vi "CTRE_PigeonIMU_Receive.vi"(11 "Device ID":u32) -> (3 "Device ID Out":u32)   [LabVIEW 2016]
uses:
  <vilib>/Rock Robotics/WPI/ThirdParty/Sensors/Pigeon IMU/CTRE_PigeonIMU_CalibrationMode.ctl
  <vilib>/Rock Robotics/WPI/ThirdParty/Sensors/Pigeon IMU/CTRE_PigeonIMU_MessageIDs.ctl
  <vilib>/Rock Robotics/WPI/ThirdParty/Sensors/Pigeon IMU/CTRE_PigeonIMU_GlobalStatus.ctl
  <vilib>/Rock Robotics/WPI/ThirdParty/Sensors/Pigeon IMU/CTRE_PigeonIMU_PigeonState.ctl
  <vilib>/Rock Robotics/WPI/ThirdParty/Sensors/Pigeon IMU/CTRE_PigeonIMU_GlobalOps.ctl
panel:
  in  "CalibrationMode":T1 items=["BootTareGryoAccel"=0, "Temperature"=1, "Magnetometer12Pt"=2, "Magnetometer360"=3, "Accelerometer"=5]
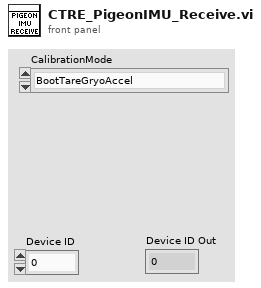
[diagram p1: front panel]
types:
  T1 = typedef "CTRE_PigeonIMU_CalibrationMode.ctl" = u16
  T2 = typedef "CTRE_PigeonIMU_MessageIDs.ctl" = u32
  T3 = typedef "CTRE_PigeonIMU_GlobalOps.ctl" = enum16{"Read For Send", "Write Error", "Get All", "Set Control Frame Rate", "Set Enable Frame Rate", "Write After Receive Fused Heading", "Write After Receive YPR", "Write After Receive Status", "Write After Receive Raw Magnetomoter", "Write After Receive Biased Magnetometer", "Write After Receive Biased Accelerometer", "Write After Receive Gyro", "Write After Receive Acceleromter Angles", "Write After Receive Startup Status", "Write After Receive Compass", "Write After Receive Quaternian", "Write After Receive AccumGyro"}
  T4 = typedef "CTRE_PigeonIMU_PigeonState.ctl" = enum16{"NoComm", "Initializing", "Ready", "UserCalibration"}
  T5 = typedef "CTRE_PigeonIMU_GlobalStatus.ctl" = cluster{"PigeonState":T4, "FusedHeading":cluster{"Heading":dbl, "Valid?":bool, "Fusing?":bool}, "YPR":cluster{"Yaw":dbl, "Pitch":dbl, "Roll":dbl}, "Compass":cluster{"Heading":dbl, "Magnitude":dbl, "Absolute Heading":dbl}, "Accelerometer":cluster{"Biased":cluster{"X":i16, "Y":i16, "Z":i16, "Norm":i16}, "Angles":cluster{"XZ Tilt":dbl, "YZ Tilt":dbl, "XY Tilt":dbl}}, "Magnetometer":cluster{"Raw":cluster{"X":i16, "Y":i16, "Z":i16}, "Biased":cluster{"X":i16, "Y":i16, "Z":i16}}, "Gyro":cluster{"X":dbl, "Y":dbl, "Z":dbl, "Norm":dbl}, "6D Quaternian":cluster{"W":dbl, "X":dbl, "Y":dbl, "Z":dbl}, "Temp. (C)":dbl, "UpTime":u32, "StartupStatus":cluster{"ResetCount":i32, "ResetFlags":i32, "FirmwareVersion":i32, "HasReset?":bool}, "Calibration":cluster{"CurrentMode":T1, "LastCalError":i32, "CalBooting?":bool}, "CAN Error":errorcluster, "AccumGyro":cluster{"X":dbl, "Y":dbl, "Z":dbl}}
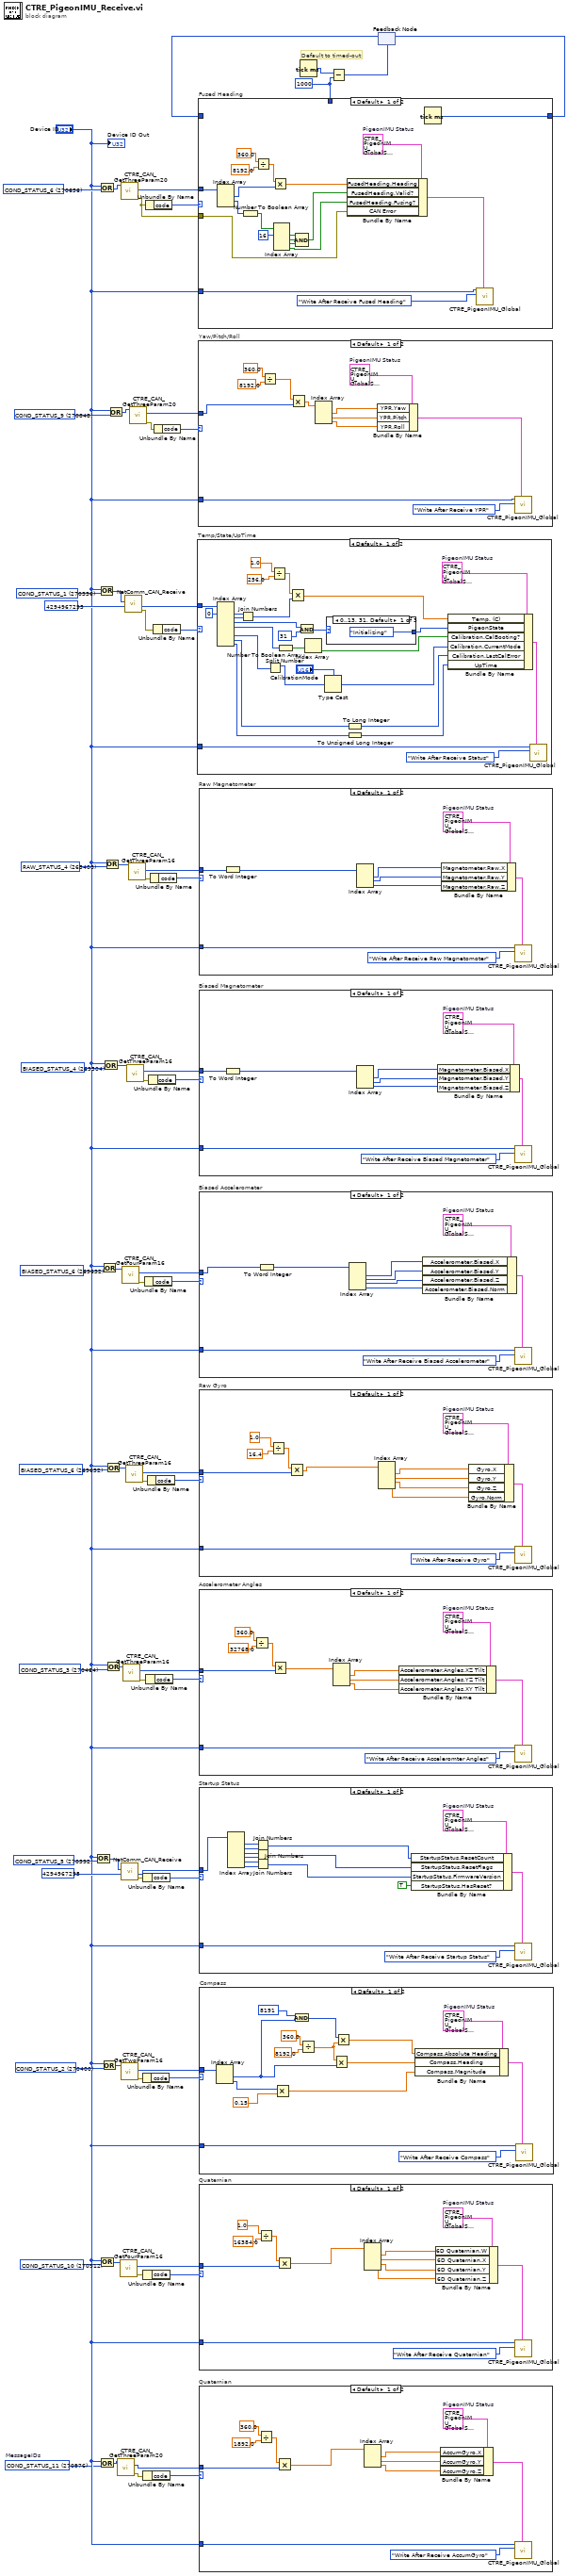
[diagram p0: block diagram]
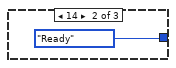
[diagram p11: hidden frame]
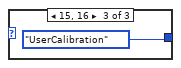
[diagram p12: hidden frame]
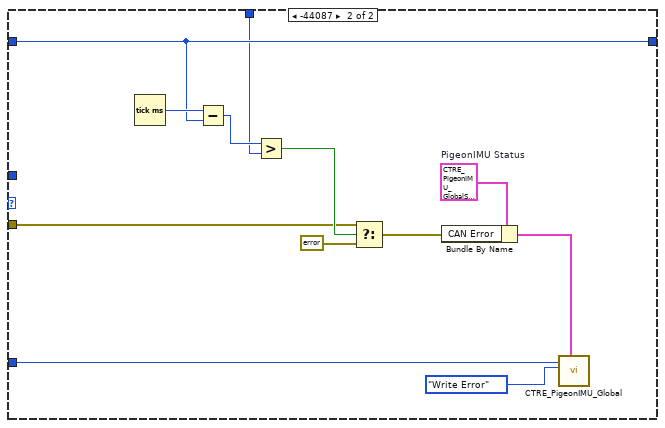
[diagram p15: hidden frame]
diagram:
  w4 = T2 270976 items=["RAW_STATUS_2"=265280, "RAW_STATUS_4"=265408, "RAW_STATUS_6"=265536, "BIASED_STATUS_2"=269376, "BIASED_STATUS_4"=269504, "BIASED_STATUS_6"=269632, "COND_STATUS_1"=270336, "COND_STATUS_2"=270400, "COND_STATUS_3"=270464, "COND_STATUS_4"=270528, "COND_STATUS_5"=270592, "COND_STATUS_6"=270656, "COND_STATUS_7"=270720, "COND_STATUS_8"=270784, "COND_STATUS_9"=270848, "COND_STATUS_10"=270912, "COND_STATUS_11"=270976, "CONTROL_1"=272384, "PARAM_REQUEST"=273408, "PARAM_RESPONSE"=273472, "PARAM_SET"=273536]  # MessageIDs
  w8 = u32 1000 ("y")
  w14 = T2 270912 items=["RAW_STATUS_2"=265280, "RAW_STATUS_4"=265408, "RAW_STATUS_6"=265536, "BIASED_STATUS_2"=269376, "BIASED_STATUS_4"=269504, "BIASED_STATUS_6"=269632, "COND_STATUS_1"=270336, "COND_STATUS_2"=270400, "COND_STATUS_3"=270464, "COND_STATUS_4"=270528, "COND_STATUS_5"=270592, "COND_STATUS_6"=270656, "COND_STATUS_7"=270720, "COND_STATUS_8"=270784, "COND_STATUS_9"=270848, "COND_STATUS_10"=270912, "CONTROL_1"=272384, "PARAM_REQUEST"=273408, "PARAM_RESPONSE"=273472, "PARAM_SET"=273536] ("MessageIDs")
  w19 = T2 270400 items=["RAW_STATUS_2"=265280, "RAW_STATUS_4"=265408, "RAW_STATUS_6"=265536, "BIASED_STATUS_2"=269376, "BIASED_STATUS_4"=269504, "BIASED_STATUS_6"=269632, "COND_STATUS_1"=270336, "COND_STATUS_2"=270400, "COND_STATUS_3"=270464, "COND_STATUS_4"=270528, "COND_STATUS_5"=270592, "COND_STATUS_6"=270656, "COND_STATUS_7"=270720, "COND_STATUS_8"=270784, "COND_STATUS_9"=270848, "COND_STATUS_10"=270912, "CONTROL_1"=272384, "PARAM_REQUEST"=273408, "PARAM_RESPONSE"=273472, "PARAM_SET"=273536] ("MessageIDs")
  w23 = T2 270592 items=["RAW_STATUS_2"=265280, "RAW_STATUS_4"=265408, "RAW_STATUS_6"=265536, "BIASED_STATUS_2"=269376, "BIASED_STATUS_4"=269504, "BIASED_STATUS_6"=269632, "COND_STATUS_1"=270336, "COND_STATUS_2"=270400, "COND_STATUS_3"=270464, "COND_STATUS_4"=270528, "COND_STATUS_5"=270592, "COND_STATUS_6"=270656, "COND_STATUS_7"=270720, "COND_STATUS_8"=270784, "COND_STATUS_9"=270848, "COND_STATUS_10"=270912, "CONTROL_1"=272384, "PARAM_REQUEST"=273408, "PARAM_RESPONSE"=273472, "PARAM_SET"=273536] ("MessageIDs")
  w31 = T2 270464 items=["RAW_STATUS_2"=265280, "RAW_STATUS_4"=265408, "RAW_STATUS_6"=265536, "BIASED_STATUS_2"=269376, "BIASED_STATUS_4"=269504, "BIASED_STATUS_6"=269632, "COND_STATUS_1"=270336, "COND_STATUS_2"=270400, "COND_STATUS_3"=270464, "COND_STATUS_4"=270528, "COND_STATUS_5"=270592, "COND_STATUS_6"=270656, "COND_STATUS_7"=270720, "COND_STATUS_8"=270784, "COND_STATUS_9"=270848, "COND_STATUS_10"=270912, "CONTROL_1"=272384, "PARAM_REQUEST"=273408, "PARAM_RESPONSE"=273472, "PARAM_SET"=273536] ("MessageIDs")
  w34 = T2 269632 items=["RAW_STATUS_2"=265280, "RAW_STATUS_4"=265408, "RAW_STATUS_6"=265536, "BIASED_STATUS_2"=269376, "BIASED_STATUS_4"=269504, "BIASED_STATUS_6"=269632, "COND_STATUS_1"=270336, "COND_STATUS_2"=270400, "COND_STATUS_3"=270464, "COND_STATUS_4"=270528, "COND_STATUS_5"=270592, "COND_STATUS_6"=270656, "COND_STATUS_7"=270720, "COND_STATUS_8"=270784, "COND_STATUS_9"=270848, "COND_STATUS_10"=270912, "CONTROL_1"=272384, "PARAM_REQUEST"=273408, "PARAM_RESPONSE"=273472, "PARAM_SET"=273536] ("MessageIDs")
  w43 = T2 269632 items=["RAW_STATUS_2"=265280, "RAW_STATUS_4"=265408, "RAW_STATUS_6"=265536, "BIASED_STATUS_2"=269376, "BIASED_STATUS_4"=269504, "BIASED_STATUS_6"=269632, "COND_STATUS_1"=270336, "COND_STATUS_2"=270400, "COND_STATUS_3"=270464, "COND_STATUS_4"=270528, "COND_STATUS_5"=270592, "COND_STATUS_6"=270656, "COND_STATUS_7"=270720, "COND_STATUS_8"=270784, "COND_STATUS_9"=270848, "COND_STATUS_10"=270912, "CONTROL_1"=272384, "PARAM_REQUEST"=273408, "PARAM_RESPONSE"=273472, "PARAM_SET"=273536] ("MessageIDs")
  w48 = T2 269504 items=["RAW_STATUS_2"=265280, "RAW_STATUS_4"=265408, "RAW_STATUS_6"=265536, "BIASED_STATUS_2"=269376, "BIASED_STATUS_4"=269504, "BIASED_STATUS_6"=269632, "COND_STATUS_1"=270336, "COND_STATUS_2"=270400, "COND_STATUS_3"=270464, "COND_STATUS_4"=270528, "COND_STATUS_5"=270592, "COND_STATUS_6"=270656, "COND_STATUS_7"=270720, "COND_STATUS_8"=270784, "COND_STATUS_9"=270848, "COND_STATUS_10"=270912, "CONTROL_1"=272384, "PARAM_REQUEST"=273408, "PARAM_RESPONSE"=273472, "PARAM_SET"=273536] ("MessageIDs")
  w49 = T2 265408 items=["RAW_STATUS_2"=265280, "RAW_STATUS_4"=265408, "RAW_STATUS_6"=265536, "BIASED_STATUS_2"=269376, "BIASED_STATUS_4"=269504, "BIASED_STATUS_6"=269632, "COND_STATUS_1"=270336, "COND_STATUS_2"=270400, "COND_STATUS_3"=270464, "COND_STATUS_4"=270528, "COND_STATUS_5"=270592, "COND_STATUS_6"=270656, "COND_STATUS_7"=270720, "COND_STATUS_8"=270784, "COND_STATUS_9"=270848, "COND_STATUS_10"=270912, "CONTROL_1"=272384, "PARAM_REQUEST"=273408, "PARAM_RESPONSE"=273472, "PARAM_SET"=273536] ("MessageIDs")
  w55 = T2 270336 items=["RAW_STATUS_2"=265280, "RAW_STATUS_4"=265408, "RAW_STATUS_6"=265536, "BIASED_STATUS_2"=269376, "BIASED_STATUS_4"=269504, "BIASED_STATUS_6"=269632, "COND_STATUS_1"=270336, "COND_STATUS_2"=270400, "COND_STATUS_3"=270464, "COND_STATUS_4"=270528, "COND_STATUS_5"=270592, "COND_STATUS_6"=270656, "COND_STATUS_7"=270720, "COND_STATUS_8"=270784, "COND_STATUS_9"=270848, "COND_STATUS_10"=270912, "CONTROL_1"=272384, "PARAM_REQUEST"=273408, "PARAM_RESPONSE"=273472, "PARAM_SET"=273536] ("MessageIDs")
  w63 = T2 270848 items=["RAW_STATUS_2"=265280, "RAW_STATUS_4"=265408, "RAW_STATUS_6"=265536, "BIASED_STATUS_2"=269376, "BIASED_STATUS_4"=269504, "BIASED_STATUS_6"=269632, "COND_STATUS_1"=270336, "COND_STATUS_2"=270400, "COND_STATUS_3"=270464, "COND_STATUS_4"=270528, "COND_STATUS_5"=270592, "COND_STATUS_6"=270656, "COND_STATUS_7"=270720, "COND_STATUS_8"=270784, "COND_STATUS_9"=270848, "COND_STATUS_10"=270912, "CONTROL_1"=272384, "PARAM_REQUEST"=273408, "PARAM_RESPONSE"=273472, "PARAM_SET"=273536] ("MessageIDs")
  w66 = T2 270656 items=["RAW_STATUS_2"=265280, "RAW_STATUS_4"=265408, "RAW_STATUS_6"=265536, "BIASED_STATUS_2"=269376, "BIASED_STATUS_4"=269504, "BIASED_STATUS_6"=269632, "COND_STATUS_1"=270336, "COND_STATUS_2"=270400, "COND_STATUS_3"=270464, "COND_STATUS_4"=270528, "COND_STATUS_5"=270592, "COND_STATUS_6"=270656, "COND_STATUS_7"=270720, "COND_STATUS_8"=270784, "COND_STATUS_9"=270848, "COND_STATUS_10"=270912, "CONTROL_1"=272384, "PARAM_REQUEST"=273408, "PARAM_RESPONSE"=273472, "PARAM_SET"=273536] ("MessageIDs")
  # "Default to timed-out"
  n1 = Or(x="Device ID", y=w23) -> (x .or. y?=w28:T2)
  n2 = Or(x="Device ID", y=w55) -> (x .or. y?=w54:T2)
  n3 = Or(x="Device ID", y=w66) -> (x .or. y?=w65:T2)
  n4 = Or(x="Device ID", y=w14) -> (x .or. y?=w15:T2)
  n5 = Or(x="Device ID", y=w4) -> (x .or. y?=w3:T2)
  n6 = Or(x="Device ID", y=w19) -> (x .or. y?=w20:T2)
  n7 = Or(x="Device ID", y=w43) -> (x .or. y?=w39:T2)
  n8 = Or(x="Device ID", y=w48) -> (x .or. y?=w47:T2)
  n9 = Or(x="Device ID", y=w49) -> (x .or. y?=w50:T2)
  n10 = Or(x="Device ID", y=w34) -> (x .or. y?=w35:T2)
  n11 = Or(x="Device ID", y=w31) -> (x .or. y?=w30:T2)
  n12 = Or(x="Device ID", y=w63) -> (x .or. y?=w64:T2)
  n13 = call <vilib>:"CTRE_CAN_GetThreeParam20.vi"("ArbID"=w3) -> ("error out"=w1:errorcluster, "3Params"=w2:i32[])  [unwired: 8 in, 1 out]
  n14 = call <vilib>:"CTRE_CAN_GetFourParam16.vi"("ArbID"=w15) -> ("error out"=w17:errorcluster, "4Params"=w13:u16[])  [unwired: 8 in, 1 out]
  n15 = call <vilib>:"CTRE_CAN_GetThreeParam20.vi"("ArbID"=w65) -> ("error out"=w7:errorcluster, "3Params"=w68:i32[])  [unwired: 8 in, 1 out]
  n16 = call <vilib>:"CTRE_CAN_GetTwoParam16.vi"("ArbID"=w20) -> ("error out"=w22:errorcluster, "2Params"=w18:u16[])  [unwired: 8 in, 1 out]
  n17 = call <vilib>:"NetComm_CAN_Receive.vi"("Message ID Mask"=u32 4294967295, "Message ID"=w28) -> ("error out"=w26:errorcluster, "Data"=w24:u8[])  [unwired: 6 in, 2 out]
  n18 = call <vilib>:"CTRE_CAN_GetFourParam16.vi"("ArbID"=w39) -> ("error out"=w40:errorcluster, "4Params"=w41:u16[])  [unwired: 8 in, 1 out]
  n19 = call <vilib>:"CTRE_CAN_GetThreeParam16.vi"("ArbID"=w30) -> ("error out"=w33:errorcluster, "3Params"=w29:u16[])  [unwired: 8 in, 1 out]
  n20 = call <vilib>:"NetComm_CAN_Receive.vi"("Message ID Mask"=u32 4294967295, "Message ID"=w54) -> ("error out"=w57:errorcluster, "Data"=w58:u8[])  [unwired: 6 in, 2 out]
  n21 = call <vilib>:"CTRE_CAN_GetThreeParam16.vi"("ArbID"=w35) -> ("error out"=w37:errorcluster, "3Params"=w36:u16[])  [unwired: 8 in, 1 out]
  n22 = call <vilib>:"CTRE_CAN_GetThreeParam16.vi"("ArbID"=w47) -> ("error out"=w46:errorcluster, "3Params"=w44:u16[])  [unwired: 8 in, 1 out]
  n23 = call <vilib>:"CTRE_CAN_GetThreeParam16.vi"("ArbID"=w50) -> ("error out"=w53:errorcluster, "3Params"=w51:u16[])  [unwired: 8 in, 1 out]
  n24 = call <vilib>:"CTRE_CAN_GetThreeParam20.vi"("ArbID"=w64) -> ("error out"=w62:errorcluster, "3Params"=w60:i32[])  [unwired: 8 in, 1 out]
  n25 = Unbundle By Name(w22) -> ("code"=w21:i32)
  n26 = Unbundle By Name(w26) -> ("code"=w25:i32)
  n27 = Unbundle By Name(w17) -> ("code"=w16:i32)
  n28 = Unbundle By Name(w1) -> ("code"=w6:i32)
  n29 = Unbundle By Name(w40) -> ("code"=w42:i32)
  n30 = Unbundle By Name(w7) -> ("code"=w67:i32)
  n31 = Unbundle By Name(w33) -> ("code"=w32:i32)
  n32 = Unbundle By Name(w37) -> ("code"=w38:i32)
  n33 = Unbundle By Name(w46) -> ("code"=w45:i32)
  n34 = Unbundle By Name(w53) -> ("code"=w52:i32)
  n35 = Unbundle By Name(w57) -> ("code"=w56:i32)
  n36 = Unbundle By Name(w62) -> ("code"=w61:i32)
  n37 = case "Temp/State/UpTime" shown="Default" w56 {
    tunnel: w58 -> [w93 _]
    tunnel: "Device ID" -> [w81 _]
    frame Default {
      w95 = T5 {"PigeonState"=enum."NoComm", "FusedHeading"={"Heading"=0.0, "Valid?"=TRUE, "Fusing?"=TRUE}, "YPR"={"Yaw"=0.0, "Pitch"=0.0, "Roll"=0.0}, "Compass"={"Heading"=0.0, "Magnitude"=0.0, "Absolute Heading"=0.0}, "Accelerometer"={"Biased"={"X"=0, "Y"=0, "Z"=0, "Norm"=0}, "Angles"={"XZ Tilt"=0.0, "YZ Tilt"=0.0, "XY Tilt"=0.0}}, "Magnetometer"={"Raw"={"X"=0, "Y"=0, "Z"=0}, "Biased"={"X"=0, "Y"=0, "Z"=0}}, "Gyro"={"X"=0.0, "Y"=0.0, "Z"=0.0, "Norm"=0.0}, "6D Quaternian"={"W"=0.0, "X"=0.0, "Y"=0.0, "Z"=0.0}, "Temp. (C)"=0.0, "UpTime"=0, "StartupStatus"={"ResetCount"=0, "ResetFlags"=0, "FirmwareVersion"=0, "HasReset?"=TRUE}, "Calibration"={"CurrentMode"=0, "LastCalError"=0, "CalBooting?"=TRUE}, "CAN Error"={"status"=FALSE, "code"=0, "source"=""}, "AccumGyro"={"X"=0.0, "Y"=0.0, "Z"=0.0}}  # PigeonIMU Status
      n38 = Index Array(array=w93, index #1=0 ("index")) -> (element #1=w92:u8, element #2=w91:u8, element #3=w90:u8, element #4=w75:u8, element #6=w72:u8, element #7=w77:u8, element #8=w78:u8)  [unwired: 7 in, 1 out]
      n39 = Join Numbers(hi=w92, lo=w91) -> ((hi.lo)=w84:u16)
      n40 = Split Number(x=w72) -> (hi(x)=w71:u8)  [unwired: 1 out]
      n41 = Divide(x=1.0, y=256.0) -> (x/y=w85:dbl)
      n42 = Number To Boolean Array(number=w75) -> (Boolean array=w74:bool[])
      n43 = Multiply(x=w85, y=w84) -> (x*y=w83:dbl)
      n44 = And(x=w90, y=u8 31) -> (x .and. y?=w89:u8)
      n45 = Index Array(array=w74) -> (element=w73:bool)  [unwired: 1 in]
      n46 = Type Cast(type="CalibrationMode", x=w71) -> (*(type *) &x=w69:T1)
      n47 = case shown="0..13, 31, Default" w89 {
        tunnel: [CTRE_PigeonIMU_PigeonState."Initializing" ("PigeonState") CTRE_PigeonIMU_PigeonState."Ready" ("PigeonState") CTRE_PigeonIMU_PigeonState."UserCalibration" ("PigeonState")] -> w88
        frame 0..13, 31, Default {
        }
        frame 14 {
        }
        frame 15, 16 {
        }
      }
      n48 = To Long Integer(number=w77) -> (32bit integer=w79:i32)
      n49 = To Unsigned Long Integer(number=w78) -> (unsigned 32bit integer=w80:u32)
      n50 = Bundle By Name(cluster=w95, "Temp. (C)"=w83, "PigeonState"=w88, "Calibration.CalBooting?"=w73, "Calibration.CurrentMode"=w69, "Calibration.LastCalError"=w79, "UpTime"=w80) -> (w94:T5)
      n51 = call <vilib>:"CTRE_PigeonIMU_Global.vi"("Write After Receive"=w94, "Operation"=CTRE_PigeonIMU_GlobalOps."Write After Receive Status", "Device ID (0)"=w81) -> ()  [unwired: 6 in, 3 out]
    }
    frame -44087 {
    }
  }
  n52 = case "Yaw/Pitch/Roll" shown="Default" w61 {
    tunnel: w60 -> [w101 _]
    tunnel: "Device ID" -> [w100 _]
    frame Default {
      w110 = T5 {"PigeonState"=enum."NoComm", "FusedHeading"={"Heading"=0.0, "Valid?"=TRUE, "Fusing?"=TRUE}, "YPR"={"Yaw"=0.0, "Pitch"=0.0, "Roll"=0.0}, "Compass"={"Heading"=0.0, "Magnitude"=0.0, "Absolute Heading"=0.0}, "Accelerometer"={"Biased"={"X"=0, "Y"=0, "Z"=0, "Norm"=0}, "Angles"={"XZ Tilt"=0.0, "YZ Tilt"=0.0, "XY Tilt"=0.0}}, "Magnetometer"={"Raw"={"X"=0, "Y"=0, "Z"=0}, "Biased"={"X"=0, "Y"=0, "Z"=0}}, "Gyro"={"X"=0.0, "Y"=0.0, "Z"=0.0, "Norm"=0.0}, "6D Quaternian"={"W"=0.0, "X"=0.0, "Y"=0.0, "Z"=0.0}, "Temp. (C)"=0.0, "UpTime"=0, "StartupStatus"={"ResetCount"=0, "ResetFlags"=0, "FirmwareVersion"=0, "HasReset?"=TRUE}, "Calibration"={"CurrentMode"=0, "LastCalError"=0, "CalBooting?"=TRUE}, "CAN Error"={"status"=FALSE, "code"=0, "source"=""}, "AccumGyro"={"X"=0.0, "Y"=0.0, "Z"=0.0}}  # PigeonIMU Status
      n53 = Divide(x=360.0, y=8192.0) -> (x/y=w106:dbl)
      n54 = Multiply(x=w106, y=w101) -> (x*y=w105:dbl[])
      n55 = Index Array(array=w105) -> (element #1=w104:dbl, element #2=w103:dbl, element #3=w102:dbl)  [unwired: 3 in]
      n56 = Bundle By Name(cluster=w110, "YPR.Yaw"=w104, "YPR.Pitch"=w103, "YPR.Roll"=w102) -> (w109:T5)
      n57 = call <vilib>:"CTRE_PigeonIMU_Global.vi"("Write After Receive"=w109, "Operation"=CTRE_PigeonIMU_GlobalOps."Write After Receive YPR", "Device ID (0)"=w100) -> ()  [unwired: 6 in, 3 out]
    }
    frame -44087 {
    }
  }
  n58 = case "Raw Magnetometer" shown="Default" w52 {
    tunnel: w51 -> [w117 _]
    tunnel: "Device ID" -> [w112 _]
    frame Default {
      w119 = T5 {"PigeonState"=enum."NoComm", "FusedHeading"={"Heading"=0.0, "Valid?"=TRUE, "Fusing?"=TRUE}, "YPR"={"Yaw"=0.0, "Pitch"=0.0, "Roll"=0.0}, "Compass"={"Heading"=0.0, "Magnitude"=0.0, "Absolute Heading"=0.0}, "Accelerometer"={"Biased"={"X"=0, "Y"=0, "Z"=0, "Norm"=0}, "Angles"={"XZ Tilt"=0.0, "YZ Tilt"=0.0, "XY Tilt"=0.0}}, "Magnetometer"={"Raw"={"X"=0, "Y"=0, "Z"=0}, "Biased"={"X"=0, "Y"=0, "Z"=0}}, "Gyro"={"X"=0.0, "Y"=0.0, "Z"=0.0, "Norm"=0.0}, "6D Quaternian"={"W"=0.0, "X"=0.0, "Y"=0.0, "Z"=0.0}, "Temp. (C)"=0.0, "UpTime"=0, "StartupStatus"={"ResetCount"=0, "ResetFlags"=0, "FirmwareVersion"=0, "HasReset?"=TRUE}, "Calibration"={"CurrentMode"=0, "LastCalError"=0, "CalBooting?"=TRUE}, "CAN Error"={"status"=FALSE, "code"=0, "source"=""}, "AccumGyro"={"X"=0.0, "Y"=0.0, "Z"=0.0}}  # PigeonIMU Status
      n59 = To Word Integer(number=w117) -> (16bit integer=w113:i16[])
      n60 = Index Array(array=w113) -> (element #1=w116:i16, element #2=w115:i16, element #3=w114:i16)  [unwired: 3 in]
      n61 = Bundle By Name(cluster=w119, "Magnetometer.Raw.X"=w116, "Magnetometer.Raw.Y"=w115, "Magnetometer.Raw.Z"=w114) -> (w118:T5)
      n62 = call <vilib>:"CTRE_PigeonIMU_Global.vi"("Write After Receive"=w118, "Operation"=CTRE_PigeonIMU_GlobalOps."Write After Receive Raw Magnetomoter", "Device ID (0)"=w112) -> ()  [unwired: 6 in, 3 out]
    }
    frame -44087 {
    }
  }
  n63 = case "Biased Magnetometer" shown="Default" w45 {
    tunnel: w44 -> [w126 _]
    tunnel: "Device ID" -> [w121 _]
    frame Default {
      w128 = T5 {"PigeonState"=enum."NoComm", "FusedHeading"={"Heading"=0.0, "Valid?"=TRUE, "Fusing?"=TRUE}, "YPR"={"Yaw"=0.0, "Pitch"=0.0, "Roll"=0.0}, "Compass"={"Heading"=0.0, "Magnitude"=0.0, "Absolute Heading"=0.0}, "Accelerometer"={"Biased"={"X"=0, "Y"=0, "Z"=0, "Norm"=0}, "Angles"={"XZ Tilt"=0.0, "YZ Tilt"=0.0, "XY Tilt"=0.0}}, "Magnetometer"={"Raw"={"X"=0, "Y"=0, "Z"=0}, "Biased"={"X"=0, "Y"=0, "Z"=0}}, "Gyro"={"X"=0.0, "Y"=0.0, "Z"=0.0, "Norm"=0.0}, "6D Quaternian"={"W"=0.0, "X"=0.0, "Y"=0.0, "Z"=0.0}, "Temp. (C)"=0.0, "UpTime"=0, "StartupStatus"={"ResetCount"=0, "ResetFlags"=0, "FirmwareVersion"=0, "HasReset?"=TRUE}, "Calibration"={"CurrentMode"=0, "LastCalError"=0, "CalBooting?"=TRUE}, "CAN Error"={"status"=FALSE, "code"=0, "source"=""}, "AccumGyro"={"X"=0.0, "Y"=0.0, "Z"=0.0}}  # PigeonIMU Status
      n64 = To Word Integer(number=w126) -> (16bit integer=w122:i16[])
      n65 = Index Array(array=w122) -> (element #1=w125:i16, element #2=w124:i16, element #3=w123:i16)  [unwired: 3 in]
      n66 = Bundle By Name(cluster=w128, "Magnetometer.Biased.X"=w125, "Magnetometer.Biased.Y"=w124, "Magnetometer.Biased.Z"=w123) -> (w127:T5)
      n67 = call <vilib>:"CTRE_PigeonIMU_Global.vi"("Write After Receive"=w127, "Operation"=CTRE_PigeonIMU_GlobalOps."Write After Receive Biased Magnetometer", "Device ID (0)"=w121) -> ()  [unwired: 6 in, 3 out]
    }
    frame -44087 {
    }
  }
  n68 = case "Biased Accelerometer" shown="Default" w42 {
    tunnel: w41 -> [w136 _]
    tunnel: "Device ID" -> [w130 _]
    frame Default {
      w138 = T5 {"PigeonState"=enum."NoComm", "FusedHeading"={"Heading"=0.0, "Valid?"=TRUE, "Fusing?"=TRUE}, "YPR"={"Yaw"=0.0, "Pitch"=0.0, "Roll"=0.0}, "Compass"={"Heading"=0.0, "Magnitude"=0.0, "Absolute Heading"=0.0}, "Accelerometer"={"Biased"={"X"=0, "Y"=0, "Z"=0, "Norm"=0}, "Angles"={"XZ Tilt"=0.0, "YZ Tilt"=0.0, "XY Tilt"=0.0}}, "Magnetometer"={"Raw"={"X"=0, "Y"=0, "Z"=0}, "Biased"={"X"=0, "Y"=0, "Z"=0}}, "Gyro"={"X"=0.0, "Y"=0.0, "Z"=0.0, "Norm"=0.0}, "6D Quaternian"={"W"=0.0, "X"=0.0, "Y"=0.0, "Z"=0.0}, "Temp. (C)"=0.0, "UpTime"=0, "StartupStatus"={"ResetCount"=0, "ResetFlags"=0, "FirmwareVersion"=0, "HasReset?"=TRUE}, "Calibration"={"CurrentMode"=0, "LastCalError"=0, "CalBooting?"=TRUE}, "CAN Error"={"status"=FALSE, "code"=0, "source"=""}, "AccumGyro"={"X"=0.0, "Y"=0.0, "Z"=0.0}}  # PigeonIMU Status
      n69 = To Word Integer(number=w136) -> (16bit integer=w131:i16[])
      n70 = Index Array(array=w131) -> (element #1=w135:i16, element #2=w134:i16, element #3=w133:i16, element #4=w132:i16)  [unwired: 4 in]
      n71 = Bundle By Name(cluster=w138, "Accelerometer.Biased.X"=w135, "Accelerometer.Biased.Y"=w134, "Accelerometer.Biased.Z"=w133, "Accelerometer.Biased.Norm"=w132) -> (w137:T5)
      n72 = call <vilib>:"CTRE_PigeonIMU_Global.vi"("Write After Receive"=w137, "Operation"=CTRE_PigeonIMU_GlobalOps."Write After Receive Biased Accelerometer", "Device ID (0)"=w130) -> ()  [unwired: 6 in, 3 out]
    }
    frame -44087 {
    }
  }
  n73 = case "Raw Gyro" shown="Default" w38 {
    tunnel: w36 -> [w146 _]
    tunnel: "Device ID" -> [w140 _]
    frame Default {
      w151 = T5 {"PigeonState"=enum."NoComm", "FusedHeading"={"Heading"=0.0, "Valid?"=TRUE, "Fusing?"=TRUE}, "YPR"={"Yaw"=0.0, "Pitch"=0.0, "Roll"=0.0}, "Compass"={"Heading"=0.0, "Magnitude"=0.0, "Absolute Heading"=0.0}, "Accelerometer"={"Biased"={"X"=0, "Y"=0, "Z"=0, "Norm"=0}, "Angles"={"XZ Tilt"=0.0, "YZ Tilt"=0.0, "XY Tilt"=0.0}}, "Magnetometer"={"Raw"={"X"=0, "Y"=0, "Z"=0}, "Biased"={"X"=0, "Y"=0, "Z"=0}}, "Gyro"={"X"=0.0, "Y"=0.0, "Z"=0.0, "Norm"=0.0}, "6D Quaternian"={"W"=0.0, "X"=0.0, "Y"=0.0, "Z"=0.0}, "Temp. (C)"=0.0, "UpTime"=0, "StartupStatus"={"ResetCount"=0, "ResetFlags"=0, "FirmwareVersion"=0, "HasReset?"=TRUE}, "Calibration"={"CurrentMode"=0, "LastCalError"=0, "CalBooting?"=TRUE}, "CAN Error"={"status"=FALSE, "code"=0, "source"=""}, "AccumGyro"={"X"=0.0, "Y"=0.0, "Z"=0.0}}  # PigeonIMU Status
      n74 = Divide(x=1.0, y=16.4) -> (x/y=w147:dbl)
      n75 = Multiply(x=w147, y=w146) -> (x*y=w145:dbl[])
      n76 = Index Array(array=w145) -> (element #1=w144:dbl, element #2=w143:dbl, element #3=w142:dbl, element #4=w141:dbl)  [unwired: 4 in]
      n77 = Bundle By Name(cluster=w151, "Gyro.X"=w144, "Gyro.Y"=w143, "Gyro.Z"=w142, "Gyro.Norm"=w141) -> (w150:T5)
      n78 = call <vilib>:"CTRE_PigeonIMU_Global.vi"("Write After Receive"=w150, "Operation"=CTRE_PigeonIMU_GlobalOps."Write After Receive Gyro", "Device ID (0)"=w140) -> ()  [unwired: 6 in, 3 out]
    }
    frame -44087 {
    }
  }
  n79 = case "Accelerometer Angles" shown="Default" w32 {
    tunnel: w29 -> [w158 _]
    tunnel: "Device ID" -> [w153 _]
    frame Default {
      w163 = T5 {"PigeonState"=enum."NoComm", "FusedHeading"={"Heading"=0.0, "Valid?"=TRUE, "Fusing?"=TRUE}, "YPR"={"Yaw"=0.0, "Pitch"=0.0, "Roll"=0.0}, "Compass"={"Heading"=0.0, "Magnitude"=0.0, "Absolute Heading"=0.0}, "Accelerometer"={"Biased"={"X"=0, "Y"=0, "Z"=0, "Norm"=0}, "Angles"={"XZ Tilt"=0.0, "YZ Tilt"=0.0, "XY Tilt"=0.0}}, "Magnetometer"={"Raw"={"X"=0, "Y"=0, "Z"=0}, "Biased"={"X"=0, "Y"=0, "Z"=0}}, "Gyro"={"X"=0.0, "Y"=0.0, "Z"=0.0, "Norm"=0.0}, "6D Quaternian"={"W"=0.0, "X"=0.0, "Y"=0.0, "Z"=0.0}, "Temp. (C)"=0.0, "UpTime"=0, "StartupStatus"={"ResetCount"=0, "ResetFlags"=0, "FirmwareVersion"=0, "HasReset?"=TRUE}, "Calibration"={"CurrentMode"=0, "LastCalError"=0, "CalBooting?"=TRUE}, "CAN Error"={"status"=FALSE, "code"=0, "source"=""}, "AccumGyro"={"X"=0.0, "Y"=0.0, "Z"=0.0}}  # PigeonIMU Status
      n80 = Divide(x=360.0, y=32768.0) -> (x/y=w161:dbl)
      n81 = Multiply(x=w161, y=w158) -> (x*y=w157:dbl[])
      n82 = Index Array(array=w157) -> (element #1=w156:dbl, element #2=w155:dbl, element #3=w154:dbl)  [unwired: 3 in]
      n83 = Bundle By Name(cluster=w163, "Accelerometer.Angles.XZ Tilt"=w156, "Accelerometer.Angles.YZ Tilt"=w155, "Accelerometer.Angles.XY Tilt"=w154) -> (w162:T5)
      n84 = call <vilib>:"CTRE_PigeonIMU_Global.vi"("Write After Receive"=w162, "Operation"=CTRE_PigeonIMU_GlobalOps."Write After Receive Acceleromter Angles", "Device ID (0)"=w153) -> ()  [unwired: 6 in, 3 out]
    }
    frame -44087 {
    }
  }
  n85 = case "Startup Status" shown="Default" w25 {
    tunnel: w24 -> [w175 _]
    tunnel: "Device ID" -> [w165 _]
    frame Default {
      w178 = T5 {"PigeonState"=enum."NoComm", "FusedHeading"={"Heading"=0.0, "Valid?"=TRUE, "Fusing?"=TRUE}, "YPR"={"Yaw"=0.0, "Pitch"=0.0, "Roll"=0.0}, "Compass"={"Heading"=0.0, "Magnitude"=0.0, "Absolute Heading"=0.0}, "Accelerometer"={"Biased"={"X"=0, "Y"=0, "Z"=0, "Norm"=0}, "Angles"={"XZ Tilt"=0.0, "YZ Tilt"=0.0, "XY Tilt"=0.0}}, "Magnetometer"={"Raw"={"X"=0, "Y"=0, "Z"=0}, "Biased"={"X"=0, "Y"=0, "Z"=0}}, "Gyro"={"X"=0.0, "Y"=0.0, "Z"=0.0, "Norm"=0.0}, "6D Quaternian"={"W"=0.0, "X"=0.0, "Y"=0.0, "Z"=0.0}, "Temp. (C)"=0.0, "UpTime"=0, "StartupStatus"={"ResetCount"=0, "ResetFlags"=0, "FirmwareVersion"=0, "HasReset?"=TRUE}, "Calibration"={"CurrentMode"=0, "LastCalError"=0, "CalBooting?"=TRUE}, "CAN Error"={"status"=FALSE, "code"=0, "source"=""}, "AccumGyro"={"X"=0.0, "Y"=0.0, "Z"=0.0}}  # PigeonIMU Status
      n86 = Index Array(array=w175) -> (element #1=w173:u8, element #2=w174:u8, element #3=w170:u8, element #4=w171:u8, element #5=w168:u8, element #6=w167:u8)  [unwired: 6 in]
      n87 = Join Numbers(hi=w173, lo=w174) -> ((hi.lo)=w172:u16)
      n88 = Join Numbers(hi=w170, lo=w171) -> ((hi.lo)=w169:u16)
      n89 = Join Numbers(hi=w168, lo=w167) -> ((hi.lo)=w166:u16)
      n90 = Bundle By Name(cluster=w178, "StartupStatus.ResetCount"=w172, "StartupStatus.ResetFlags"=w169, "StartupStatus.FirmwareVersion"=w166, "StartupStatus.HasReset?"=TRUE) -> (w177:T5)
      n91 = call <vilib>:"CTRE_PigeonIMU_Global.vi"("Write After Receive"=w177, "Operation"=CTRE_PigeonIMU_GlobalOps."Write After Receive Startup Status", "Device ID (0)"=w165) -> ()  [unwired: 6 in, 3 out]
    }
    frame -44087 {
    }
  }
  n92 = case "Quaternian" shown="Default" w16 {
    tunnel: w13 -> [w186 _]
    tunnel: "Device ID" -> [w180 _]
    frame Default {
      w191 = T5 {"PigeonState"=enum."NoComm", "FusedHeading"={"Heading"=0.0, "Valid?"=TRUE, "Fusing?"=TRUE}, "YPR"={"Yaw"=0.0, "Pitch"=0.0, "Roll"=0.0}, "Compass"={"Heading"=0.0, "Magnitude"=0.0, "Absolute Heading"=0.0}, "Accelerometer"={"Biased"={"X"=0, "Y"=0, "Z"=0, "Norm"=0}, "Angles"={"XZ Tilt"=0.0, "YZ Tilt"=0.0, "XY Tilt"=0.0}}, "Magnetometer"={"Raw"={"X"=0, "Y"=0, "Z"=0}, "Biased"={"X"=0, "Y"=0, "Z"=0}}, "Gyro"={"X"=0.0, "Y"=0.0, "Z"=0.0, "Norm"=0.0}, "6D Quaternian"={"W"=0.0, "X"=0.0, "Y"=0.0, "Z"=0.0}, "Temp. (C)"=0.0, "UpTime"=0, "StartupStatus"={"ResetCount"=0, "ResetFlags"=0, "FirmwareVersion"=0, "HasReset?"=TRUE}, "Calibration"={"CurrentMode"=0, "LastCalError"=0, "CalBooting?"=TRUE}, "CAN Error"={"status"=FALSE, "code"=0, "source"=""}, "AccumGyro"={"X"=0.0, "Y"=0.0, "Z"=0.0}}  # PigeonIMU Status
      n93 = Divide(x=1.0, y=16384.0) -> (x/y=w189:dbl)
      n94 = Multiply(x=w189, y=w186) -> (x*y=w185:dbl[])
      n95 = Index Array(array=w185) -> (element #1=w184:dbl, element #2=w183:dbl, element #3=w182:dbl, element #4=w181:dbl)  [unwired: 4 in]
      n96 = Bundle By Name(cluster=w191, "6D Quaternian.W"=w184, "6D Quaternian.X"=w183, "6D Quaternian.Y"=w182, "6D Quaternian.Z"=w181) -> (w190:T5)
      n97 = call <vilib>:"CTRE_PigeonIMU_Global.vi"("Write After Receive"=w190, "Operation"=CTRE_PigeonIMU_GlobalOps."Write After Receive Quaternian", "Device ID (0)"=w180) -> ()  [unwired: 6 in, 3 out]
    }
    frame -44087 {
    }
  }
  n98 = case "Quaternian" shown="Default" w6 {
    tunnel: w2 -> [w198 _]
    tunnel: "Device ID" -> [w193 _]
    frame Default {
      w203 = T5 {"PigeonState"=enum."NoComm", "FusedHeading"={"Heading"=0.0, "Valid?"=TRUE, "Fusing?"=TRUE}, "YPR"={"Yaw"=0.0, "Pitch"=0.0, "Roll"=0.0}, "Compass"={"Heading"=0.0, "Magnitude"=0.0, "Absolute Heading"=0.0}, "Accelerometer"={"Biased"={"X"=0, "Y"=0, "Z"=0, "Norm"=0}, "Angles"={"XZ Tilt"=0.0, "YZ Tilt"=0.0, "XY Tilt"=0.0}}, "Magnetometer"={"Raw"={"X"=0, "Y"=0, "Z"=0}, "Biased"={"X"=0, "Y"=0, "Z"=0}}, "Gyro"={"X"=0.0, "Y"=0.0, "Z"=0.0, "Norm"=0.0}, "6D Quaternian"={"W"=0.0, "X"=0.0, "Y"=0.0, "Z"=0.0}, "Temp. (C)"=0.0, "UpTime"=0, "StartupStatus"={"ResetCount"=0, "ResetFlags"=0, "FirmwareVersion"=0, "HasReset?"=TRUE}, "Calibration"={"CurrentMode"=0, "LastCalError"=0, "CalBooting?"=TRUE}, "CAN Error"={"status"=FALSE, "code"=0, "source"=""}, "AccumGyro"={"X"=0.0, "Y"=0.0, "Z"=0.0}}  # PigeonIMU Status
      n99 = Divide(x=360.0, y=1892.0) -> (x/y=w201:dbl)
      n100 = Multiply(x=w201, y=w198) -> (x*y=w197:dbl[])
      n101 = Index Array(array=w197) -> (element #1=w196:dbl, element #2=w195:dbl, element #3=w194:dbl)  [unwired: 3 in]
      n102 = Bundle By Name(cluster=w203, "AccumGyro.X"=w196, "AccumGyro.Y"=w195, "AccumGyro.Z"=w194) -> (w202:T5)
      n103 = call <vilib>:"CTRE_PigeonIMU_Global.vi"("Write After Receive"=w202, "Operation"=CTRE_PigeonIMU_GlobalOps."Write After Receive AccumGyro", "Device ID (0)"=w193) -> ()  [unwired: 6 in, 3 out]
    }
    frame -44087 {
    }
  }
  n104 = case "Compass" shown="Default" w21 {
    tunnel: w18 -> [w215 _]
    tunnel: "Device ID" -> [w211 _]
    frame Default {
      w219 = T5 {"PigeonState"=enum."NoComm", "FusedHeading"={"Heading"=0.0, "Valid?"=TRUE, "Fusing?"=TRUE}, "YPR"={"Yaw"=0.0, "Pitch"=0.0, "Roll"=0.0}, "Compass"={"Heading"=0.0, "Magnitude"=0.0, "Absolute Heading"=0.0}, "Accelerometer"={"Biased"={"X"=0, "Y"=0, "Z"=0, "Norm"=0}, "Angles"={"XZ Tilt"=0.0, "YZ Tilt"=0.0, "XY Tilt"=0.0}}, "Magnetometer"={"Raw"={"X"=0, "Y"=0, "Z"=0}, "Biased"={"X"=0, "Y"=0, "Z"=0}}, "Gyro"={"X"=0.0, "Y"=0.0, "Z"=0.0, "Norm"=0.0}, "6D Quaternian"={"W"=0.0, "X"=0.0, "Y"=0.0, "Z"=0.0}, "Temp. (C)"=0.0, "UpTime"=0, "StartupStatus"={"ResetCount"=0, "ResetFlags"=0, "FirmwareVersion"=0, "HasReset?"=TRUE}, "Calibration"={"CurrentMode"=0, "LastCalError"=0, "CalBooting?"=TRUE}, "CAN Error"={"status"=FALSE, "code"=0, "source"=""}, "AccumGyro"={"X"=0.0, "Y"=0.0, "Z"=0.0}}  # PigeonIMU Status
      n105 = Index Array(array=w215) -> (element #1=w208:u16, element #2=w214:u16)  [unwired: 2 in]
      n106 = Multiply(x=w214, y=0.15) -> (x*y=w212:dbl)
      n107 = And(x=u16 8191, y=w208) -> (x .and. y?=w206:u16)
      n108 = Divide(x=360.0, y=8192.0) -> (x/y=w209:dbl)
      n109 = Multiply(x=w209, y=w208) -> (x*y=w210:dbl)
      n110 = Multiply(x=w206, y=w209) -> (x*y=w205:dbl)
      n111 = Bundle By Name(cluster=w219, "Compass.Absolute Heading"=w205, "Compass.Heading"=w210, "Compass.Magnitude"=w212) -> (w218:T5)
      n112 = call <vilib>:"CTRE_PigeonIMU_Global.vi"("Write After Receive"=w218, "Operation"=CTRE_PigeonIMU_GlobalOps."Write After Receive Compass", "Device ID (0)"=w211) -> ()  [unwired: 6 in, 3 out]
    }
    frame -44087 {
    }
  }
  n113 = Tick Count (ms)() -> (millisecond timer value=w12:u32)
  n114 = Subtract(x=w12, y=w8) -> (x-y=w11:u32)
  n115 = feedback #1(w11) -> (w10:u32)
  n116 = case "Fused Heading" shown="Default" w67 {
    tunnel: w68 -> [w240 _]
    tunnel: w10 -> [_ w250]
    tunnel: [w223 w250] -> w9
    tunnel: w8 -> [_ w249]
    tunnel: w7 -> [w222 w247]
    tunnel: "Device ID" -> [w221 w241]
    frame Default {
      w239 = T5 {"PigeonState"=enum."NoComm", "FusedHeading"={"Heading"=0.0, "Valid?"=TRUE, "Fusing?"=TRUE}, "YPR"={"Yaw"=0.0, "Pitch"=0.0, "Roll"=0.0}, "Compass"={"Heading"=0.0, "Magnitude"=0.0, "Absolute Heading"=0.0}, "Accelerometer"={"Biased"={"X"=0, "Y"=0, "Z"=0, "Norm"=0}, "Angles"={"XZ Tilt"=0.0, "YZ Tilt"=0.0, "XY Tilt"=0.0}}, "Magnetometer"={"Raw"={"X"=0, "Y"=0, "Z"=0}, "Biased"={"X"=0, "Y"=0, "Z"=0}}, "Gyro"={"X"=0.0, "Y"=0.0, "Z"=0.0, "Norm"=0.0}, "6D Quaternian"={"W"=0.0, "X"=0.0, "Y"=0.0, "Z"=0.0}, "Temp. (C)"=0.0, "UpTime"=0, "StartupStatus"={"ResetCount"=0, "ResetFlags"=0, "FirmwareVersion"=0, "HasReset?"=TRUE}, "Calibration"={"CurrentMode"=0, "LastCalError"=0, "CalBooting?"=TRUE}, "CAN Error"={"status"=FALSE, "code"=0, "source"=""}, "AccumGyro"={"X"=0.0, "Y"=0.0, "Z"=0.0}}  # PigeonIMU Status
      n117 = Index Array(array=w240) -> (element #1=w235:i32, element #2=w233:i32)  [unwired: 3 in, 1 out]
      n118 = Number To Boolean Array(number=w233) -> (Boolean array=w232:bool[])
      n119 = Divide(x=360.0, y=8192.0) -> (x/y=w236:dbl)
      n120 = Multiply(x=w236, y=w235) -> (x*y=w234:dbl)
      n121 = Index Array(array=w232, index #1=16 ("index")) -> (element #1=w230:bool, element #2=w229:bool, element #3=w228:bool, element #4=w226:bool)  [unwired: 3 in]
      n122 = Compound Arithmetic op=AND(w230, w229, w228) -> (w227:bool)
      n123 = Bundle By Name(cluster=w239, "FusedHeading.Heading"=w234, "FusedHeading.Valid?"=w227, "FusedHeading.Fusing?"=w226, "CAN Error"=w222) -> (w224:T5)
      n124 = Tick Count (ms)() -> (millisecond timer value=w223:u32)
      n125 = call <vilib>:"CTRE_PigeonIMU_Global.vi"("Write After Receive"=w224, "Operation"=CTRE_PigeonIMU_GlobalOps."Write After Receive Fused Heading", "Device ID (0)"=w221) -> ()  [unwired: 6 in, 3 out]
    }
    frame -44087 {
      w244 = T5 {"PigeonState"=enum."NoComm", "FusedHeading"={"Heading"=0.0, "Valid?"=TRUE, "Fusing?"=TRUE}, "YPR"={"Yaw"=0.0, "Pitch"=0.0, "Roll"=0.0}, "Compass"={"Heading"=0.0, "Magnitude"=0.0, "Absolute Heading"=0.0}, "Accelerometer"={"Biased"={"X"=0, "Y"=0, "Z"=0, "Norm"=0}, "Angles"={"XZ Tilt"=0.0, "YZ Tilt"=0.0, "XY Tilt"=0.0}}, "Magnetometer"={"Raw"={"X"=0, "Y"=0, "Z"=0}, "Biased"={"X"=0, "Y"=0, "Z"=0}}, "Gyro"={"X"=0.0, "Y"=0.0, "Z"=0.0, "Norm"=0.0}, "6D Quaternian"={"W"=0.0, "X"=0.0, "Y"=0.0, "Z"=0.0}, "Temp. (C)"=0.0, "UpTime"=0, "StartupStatus"={"ResetCount"=0, "ResetFlags"=0, "FirmwareVersion"=0, "HasReset?"=TRUE}, "Calibration"={"CurrentMode"=0, "LastCalError"=0, "CalBooting?"=TRUE}, "CAN Error"={"status"=FALSE, "code"=0, "source"=""}, "AccumGyro"={"X"=0.0, "Y"=0.0, "Z"=0.0}}  # PigeonIMU Status
      n126 = Tick Count (ms)() -> (millisecond timer value=w251:u32)
      n127 = Subtract(x=w251, y=w250) -> (x-y=w252:u32)
      n128 = Greater?(x=w252, y=w249) -> (0:w248:bool)
      n129 = Select(t=w247, s=w248, f=errorcluster {"status"=FALSE, "code"=0, "source"=""}) -> (s? t:f=w245:errorcluster)
      n130 = Bundle By Name(cluster=w244, "CAN Error"=w245) -> (w243:T5)
      n131 = call <vilib>:"CTRE_PigeonIMU_Global.vi"("Write After Receive"=w243, "Operation"=CTRE_PigeonIMU_GlobalOps."Write Error", "Device ID (0)"=w241) -> ()  [unwired: 6 in, 3 out]
    }
  }
  n132 = feedback-in #1(w9) -> ()
  "Device ID Out" <- "Device ID"
